vi "Append Text Table to Report.vi"(0 "report in":refnum<class "NI_report.lvclass">, 1 "column width (1)":dbl=1.0 format="%.2f", 2 "measurement system":u16(ring)=2 caption="measurement system for column width (Default)" items=["US", "Metric", "Default"], 3 "MS Office parameters":T2, 5 "column headers":string[](array[string]), 7 "row headers":string[](array[string]), 9 "text data":string[][](array[string]), 11 "error in (no error)":errorcluster, 13 "separate page? (NO)":bool, 14 "show grid lines (YES)":bool=TRUE) -> (4 "report out":refnum<class "NI_report.lvclass">, 8 "range (wd) - start (xl)":T1, 10 "end (xl)":cluster{"row (xl) ":i32, "col (xl) ":i32}, 15 "error out":errorcluster)   [LabVIEW 2017, in "NI_report.lvclass"]
doc: "Appends a 2D array to a report as a table with the given column width. You can use this polymorphic VI to append an array of strings or numbers. The data type you wire to the <B>text data</B> input determines the polymorphic instance to use."
uses:
  <vilib>/Utility/NIReport.llb/NI_report.lvclass
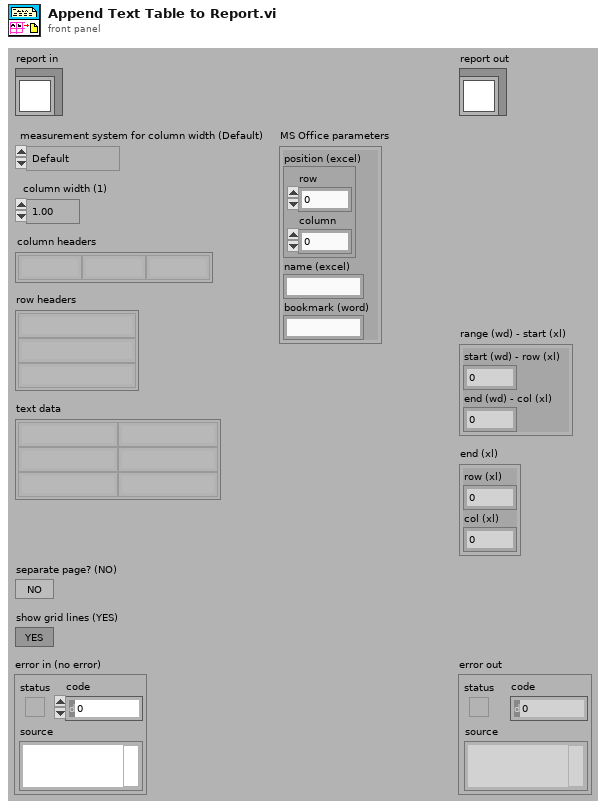
[diagram p1: front panel]
types:
  T1 = cluster{"start (wd) - row (xl) ":i32, "end (wd) - col (xl) ":i32}
  T2 = cluster{"position (excel)":cluster{"row":i32, "column":i32}, "name (excel)":string, "bookmark (word)":string}
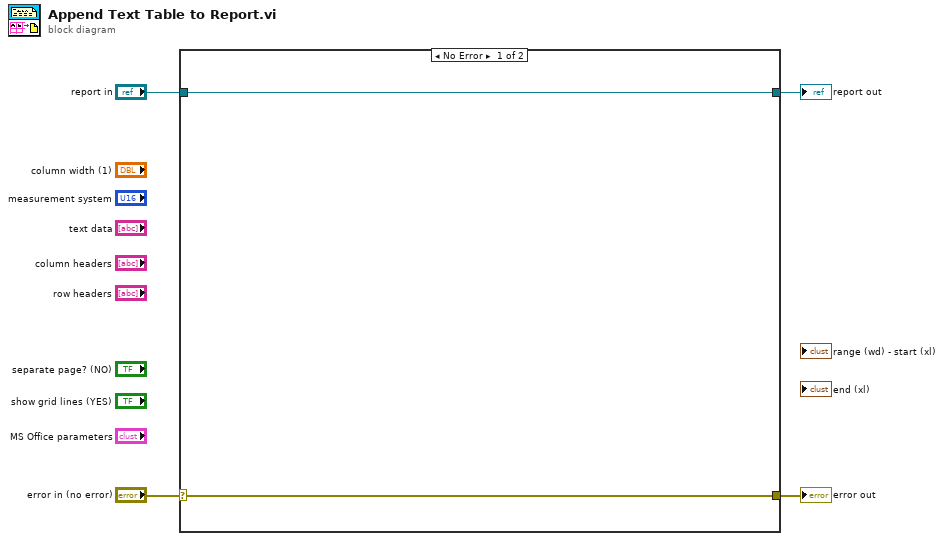
[diagram p0: block diagram]
diagram:
  n1 = case shown="No Error" "error in (no error)" {
    selector: "error in (no error)" -> [w6 w8]
    tunnel: [w6 w8] -> w3
    tunnel: [w5 w7] -> w1
    tunnel: "report in" -> [w5 w7]
    frame No Error {
    }
    frame Error {
    }
  }
  "error out" <- w3
  "report out" <- w1
